vi "Get Channel Indices.vi"(8 "error in (no error)":errorcluster, 11 "Control Experiment":refnum<class "SMO.Control Experiment.lvclass">) -> (0 "error out":errorcluster, 2 "Indices":T1, 3 "Control Experiment out":refnum<class "SMO.Control Experiment.lvclass">)   [LabVIEW 2019, in "SMO.Control Experiment.lvclass"]
uses:
  SMO.Control Experiment.lvclass
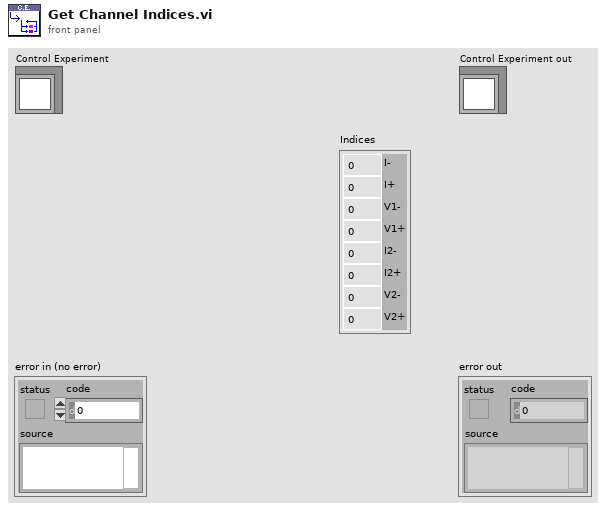
[diagram p1: front panel]
types:
  T1 = cluster{"I-":i32, "I+":i32, "V1-":i32, "V1+":i32, "I2-":i32, "I2+":i32, "V2-":i32, "V2+":i32}
  T2 = cluster{"[0]":i32, "[1]":i32, "[2]":i32, "[3]":i32, "[4]":i32, "[5]":i32}
  T3 = typedef "SMO.Control Experiment.lvclass/Wiring Description--cluster.ctl" = cluster{"AI":cluster{"Channel":u32, "Gain":dbl}, "Device":cluster{"Electrode":string, "Label":string, "Type":string}, "KH":cluster{"Channel":string, "Configuration":string, "Gain":u32, "Shunt Resistor":u32}, "AO":cluster{"Channel":u32, "Gain":dbl}}[]
  T4 = typedef "Dictionary Object RefNum__ogtk.ctl" = refnum<k1>
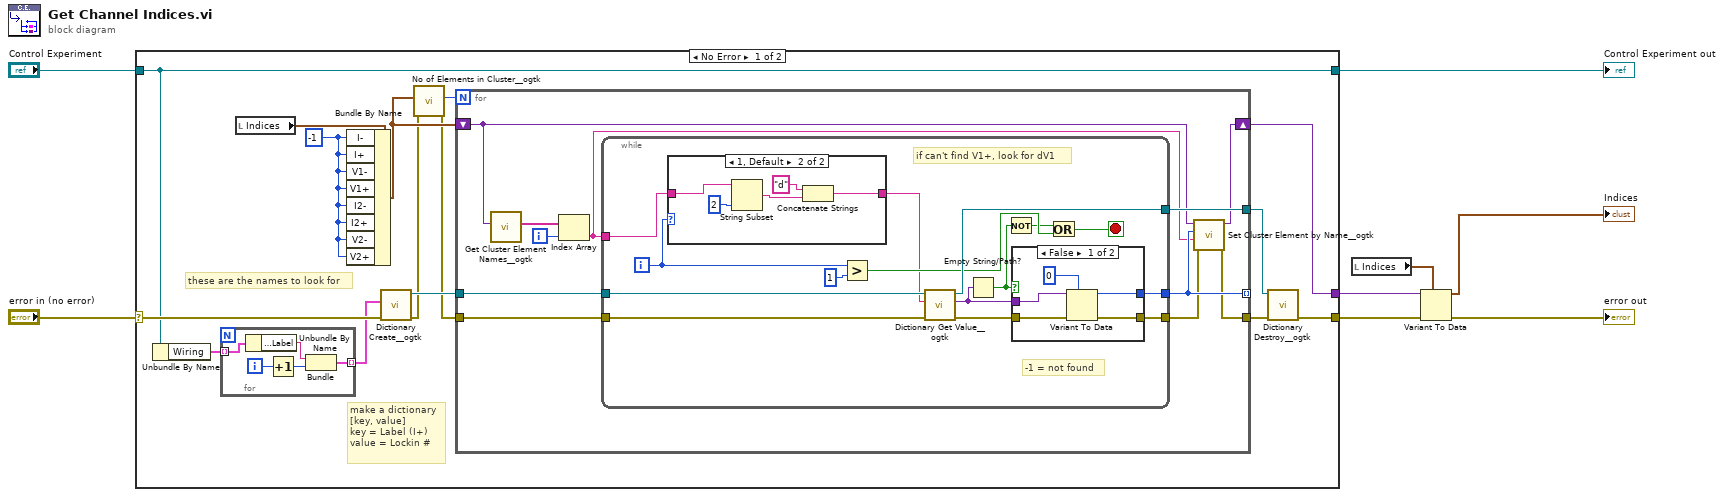
[diagram p0: block diagram]
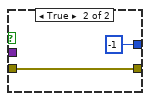
[diagram p3: hidden frame]
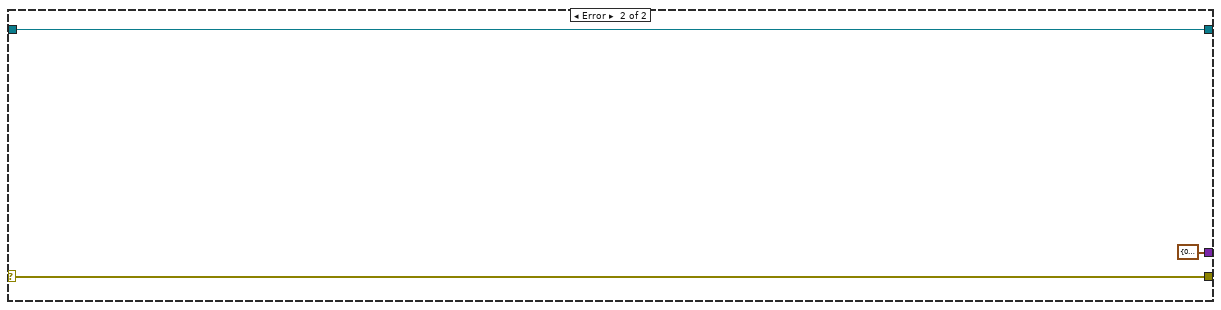
[diagram p4: hidden frame]
diagram:
  n1 = case shown="No Error" "error in (no error)" {
    selector: "error in (no error)" -> [w23 w70]
    tunnel: [w19 w70] -> w4
    tunnel: [w17 w69] -> w2
    tunnel: "Control Experiment" -> [w17 w69]
    tunnel: [w9 T2 {"[0]"=0, "[1]"=0, "[2]"=0, "[3]"=0, "[4]"=0, "[5]"=0}] -> w6
    frame No Error {
      w13 = -1 ("I-")
      # "these are the names to look for"
      # "make a dictionary\n[key, value]\nkey = Label (I+)\nvalue = Lockin #"
      n2 = Unbundle By Name(w17) -> ("Wiring"=w18:T3)
      n3 = for {
        tunnel: w18 -> [w65] mode=indexing
        tunnel: [w67] -> w14 mode=indexing
        i -> [w66]
        n4 = Unbundle By Name(w65) -> ("Device.Label"=w63:string)
        n5 = Increment(x=w66) -> (x+1=w64:i32)
        n6 = Bundle("Label"=w63, w64) -> (w67:cluster{"Label":string, i32})  [unwired: 1 in]
      }
      n7 = local read "Indices"() -> (w15:T1)
      n8 = Bundle By Name(cluster=w15, "I-"=w13, "I+"=w13, "V1-"=w13, "V1+"=w13, "I2-"=w13, "I2+"=w13, "V2-"=w13, "V2+"=w13) -> (w12:T1)
      n9 = call <userlib>:"Dictionary Create__ogtk.vi"("error in (no error)"=w23, "initial dictionary (empty)"=w14) -> ("error out"=w11:errorcluster, "dictionary out"=w22:T4)  [unwired: 8 in]
      n10 = call <userlib>:"No of Elements in Cluster__ogtk.vi"("error in (no error)"=w11, "Cluster"=w12) -> ("error out"=w10:errorcluster, "Number of Elements"=w16:u16)  [unwired: 8 in]
      n11 = for {
        N: w16 -> [_]
        tunnel: w22 -> [w34]
        tunnel: [w33] -> w21
        tunnel: w10 -> [w32]
        tunnel: [w24] -> w20
        tunnel: [w31] -> _ mode=indexing
        shift-right: [w27] -> w9
        shift-left: w12 -> [w30]
        i -> [w28]
        n12 = call <userlib>:"Get Cluster Element Names__ogtk.vi"("Cluster"=w30) -> ("Element Names"=w29:string[])  [unwired: 9 in, 1 out]
        n13 = Index Array(array=w29, index=w28) -> (element=w26:string)
        n14 = while {
          tunnel: [w46] -> w31
          tunnel: w26 -> [w36]
          tunnel: w34 -> [w49]
          tunnel: [w48] -> w33
          tunnel: w32 -> [w47]
          tunnel: [w44] -> w25
          i -> [w38]
          stop <- w42 stop-if-true
          # "-1 = not found"
          # "if can't find V1+, look for dV1"
          n15 = case shown="1, Default" w38 {
            tunnel: [w50 w53] -> w37
            tunnel: w36 -> [w50 w55]
            frame 0 {
            }
            frame 1, Default {
              n16 = String Subset(string=w55, length (rest)=2 ("length (rest)")) -> (substring=w52:string)  [unwired: 1 in]
              n17 = Concatenate Strings("d" ("string"), w52) -> (w53:string)
            }
          }
          n18 = Greater?(x=w38, y=1) -> (0:w39:bool)
          n19 = call <userlib>:"Dictionary Get Value__ogtk.vi"("error in"=w47, "key"=w37, "dictionary"=w49) -> ("error out"=w45:errorcluster, "value"=w43:variant, "dictionary out"=w48:T4)  [unwired: 5 in, 1 out]
          n20 = Empty String/Path?(string/path=w43) -> (empty?=w41:bool)
          n21 = Not(x=w41) -> (.not. x?=w35:bool)
          n22 = case shown="False" w41 {
            tunnel: [w60 w61] -> w44
            tunnel: [w59 -1 ("x+1")] -> w46
            tunnel: w43 -> [w58 _]
            tunnel: w45 -> [w56 w61]
            frame False {
              n23 = Variant To Data(error in=w56, type=0 ("x+1"), Variant=w58) -> (data=w59:i32, error out=w60:errorcluster)
            }
            frame True {
            }
          }
          n24 = Or(x=w35, y=w39) -> (x .or. y?=w42:bool)
        }
        n25 = call <userlib>:"Set Cluster Element by Name__ogtk.vi"("error in (no error)"=w25, "Element Name (\"\": New Element Data Name)"=w26, "New Element Value"=w31, "Cluster"=w30) -> ("error out"=w24:errorcluster, "VCluster out"=w27:variant)  [unwired: 5 in, 1 out]
      }
      n26 = call <userlib>:"Dictionary Destroy__ogtk.vi"("error in (no error)"=w20, "dictionary"=w21) -> ("error out"=w19:errorcluster)  [unwired: 9 in]
    }
    frame Error {
    }
  }
  "Control Experiment out" <- w2
  n27 = local read "Indices"() -> (w5:T1)
  n28 = Variant To Data(error in=w4, type=w5, Variant=w6) -> (data=→"Indices":T1, error out=→"error out":errorcluster)
